vi "PassLenghtCriteria.vi"(8 "error in (no error)":errorcluster, 10 "Point":dbl[](array[numeric]), 11 "PassObjective in":refnum<class "PassObjective.lvclass">) -> (0 "error out":errorcluster, 2 "Evaluation":dbl, 3 "PassObjective out":refnum<class "PassObjective.lvclass">)   [LabVIEW 2023, in "PassObjective.lvclass"]
uses:
  PassObjective.lvclass
  PassObjective.lvclass/PassObjective.ctl
  Game_class/Game.lvclass/Game.ctl
  Object_class/Object.lvclass/Object.ctl
  Game_class/Read BallRef.vi
  Object_class/Read position(x,y).vi
  Ball_class/Ball.lvclass
  C:/Users/ebert/Documents/codes/SSL/repo/SSL_AI/Object_class/Object.lvclass
  Utilities_class/Utilities.lvclass
  Game_class/Game.lvclass
panel:
  in  "lower limit":dbl
  in  "upper limit":dbl
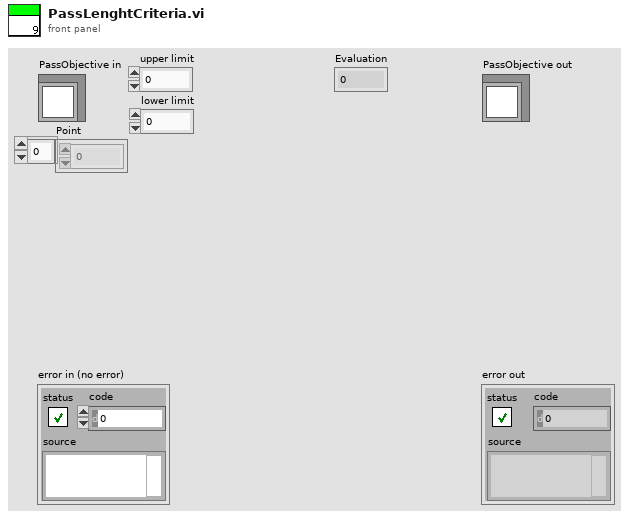
[diagram p1: front panel]
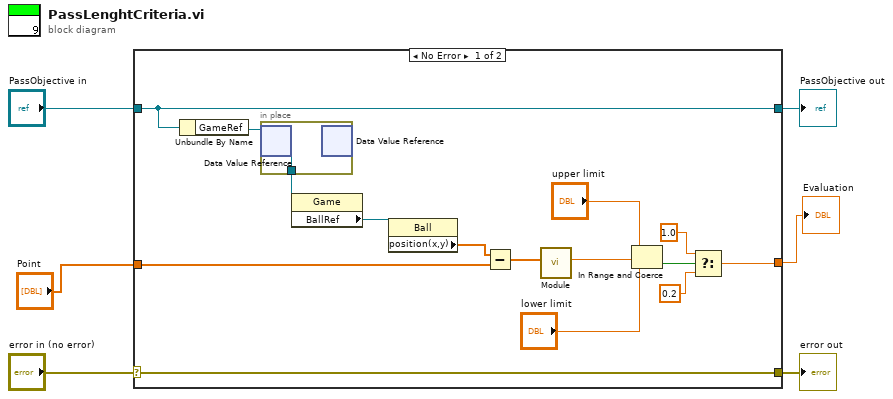
[diagram p0: block diagram]
diagram:
  n1 = case shown="No Error" "error in (no error)" {
    selector: "error in (no error)" -> [w21 w24]
    tunnel: [w21 w24] -> w5
    tunnel: [w20 w23] -> w3
    tunnel: "PassObjective in" -> [w20 w23]
    tunnel: "Point" -> [w15 _]
    tunnel: [w7 _] -> w1
    frame No Error {
      n2 = Unbundle By Name(w20) -> ("GameRef"=w19:refnum<data-value>)
      n3 = in-place {
        in-place-border: [w22] -> w18
        n4 = in-place-dvr #1(w19) -> (w22:refnum<class "Game.lvclass">)  [unwired: 1 out]
        n5 = in-place-dvr #1() -> ()  [unwired: 1 in, 2 out]
      }
      n6 = property class="Game"(reference=w18) -> ("BallRef"=w17:refnum<class "Ball.lvclass">)  [unwired: 1 in, 2 out]
      n7 = property class="Ball"(reference=w17) -> ("position(x,y)"=w16:dbl[])  [unwired: 1 in, 2 out]
      n8 = Subtract(x=w16, y=w15) -> (x-y=w14:dbl[])
      n9 = call "Module.vi"("2D vector"=w14) -> ("Modulo"=w11:dbl)  [unwired: 8 in, 2 out]
      n10 = In Range and Coerce(upper limit="upper limit", x=w11, lower limit="lower limit") -> (In Range?=w10:bool)  [unwired: 1 out]
      n11 = Select(t=1.0, s=w10, f=0.2) -> (s? t:f=w7:dbl)
    }
    frame Error {
    }
  }
  "error out" <- w5
  "PassObjective out" <- w3
  "Evaluation" <- w1
